vi "Vision_Init.vi"(10 "Front Panel.WinBounds":T1, 11 "Refnum in":T2="cam1") -> (0 "error out":errorcluster, 1 "Image (duplicate)":T4, 2 "Object Tracking Session Out":T5, 3 "Refnum out":T2, 4 "Center Point":T3)   [LabVIEW 2017]
doc: "This VI configures a USB camera for frame grabbing, and sets up the first image with the Traditional MeanShift tracking algorithm. Select the center point of the image, and place a rectangle around the region of interest to set up tracking."
uses:
  <vilib>/userdefined/High Color/IMAQdx.ctl
  <vilib>/vision/Tracking.llb/IMAQ Object Tracking Session.ctl
  <vilib>/vision/Image Controls.llb/IMAQ Image.ctl
  <vilib>/Utility/miscctls.llb/LVRectTypeDef.ctl
  <vilib>/vision/driver/NI_Vision_Acquisition_Software.lvlib
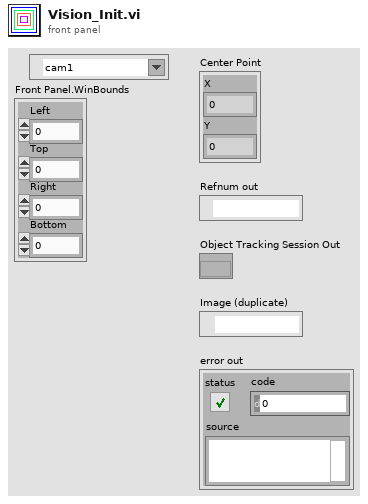
[diagram p1: front panel]
types:
  T1 = typedef "LVRectTypeDef.ctl" = cluster{"Left":i16, "Top":i16, "Right":i16, "Bottom":i16}
  T2 = typedef "IMAQdx.ctl" = refnum<k21>
  T3 = typedef "IMAQ Point" = cluster{"X":sgl, "Y":sgl}
  T4 = typedef "IMAQ Image.ctl" = refnum<image>
  T5 = typedef "IMAQ Object Tracking Session.ctl" = refnum<k20>
  T6 = typedef "Image Type" = u32
  T7 = cluster{"Number of Histogram Bins":i32, "Blending Parameter (%)":dbl, "Maximum Iterations":i32}
  T8 = typedef "ROI Descriptor" = cluster{"Global Rectangle":i32[], "Contours":cluster{"ID":enum32{"External", "Internal"}, "Type":u32, "Coordinates":i32[]}[]}
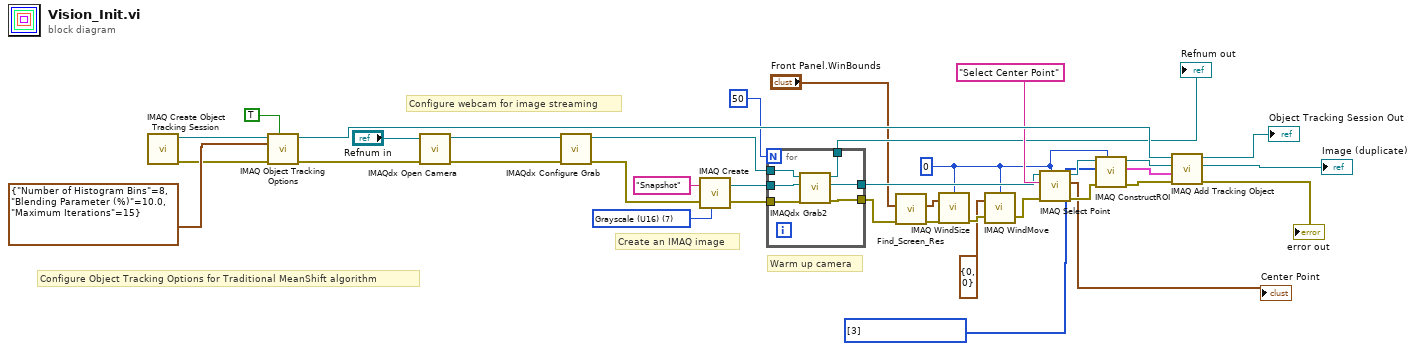
[diagram p0: block diagram]
diagram:
  w2 = 0 ("Window Number")
  w32 = u32[] [3] items=["No Selection", "Point", "Line", "Rectangle", "Oval", "Polygon", "Freehand Region", "Annulus", "Zoom", "Pan", "Broken Line", "Freehand Line", "Rotated Rectangle"] ("Tools")
  w15 = T6 7 items=["Grayscale (U8)", "Grayscale (I16)", "Grayscale (SGL)", "Complex (CSG)", "RGB (U32)", "HSL (U32)", "RGB (U64)", "Grayscale (U16)"] ("Image Type")
  # "Warm up camera"
  # "Create an IMAQ image"
  # "Configure webcam for image streaming"
  # "Configure Object Tracking Options for Traditional MeanShift algorithm"
  n1 = call "IMAQ Create Object Tracking Session"() -> ("error out"=w12:errorcluster, "Object Tracking Session"=w10:T5)  [unwired: 1 in, 9 out]
  n2 = call-poly "IMAQ Object Tracking Options"("Get/Set (Get)"=TRUE, "error in (no error)"=w12, "Mean Shift Options in"=T7 {"Number of Histogram Bins"=8, "Blending Parameter (%)"=10.0, "Maximum Iterations"=15}, "Object Tracking Session In"=w10) -> ("error out"=w16:errorcluster, "Object Tracking Session Out"=w37:T5)  [unwired: 5 in, 1 out]
  n3 = call <vilib>:"IMAQdx Open Camera.vi"("error in"=w16, "Session In"="Refnum in") -> ("error out"=w18:errorcluster, "Session Out"=w17:T2)  [unwired: 8 in]
  n4 = call <vilib>:"IMAQdx Configure Grab.vi"("error in"=w18, "Session In"=w17) -> ("error out"=w19:errorcluster, "Session Out"=w21:T2)  [unwired: 8 in]
  n5 = call "IMAQ Create"("Image Name"="Snapshot", "Image Type"=w15, "error in (no error)"=w19) -> ("New Image"=w22:T4, "error out"=w23:errorcluster)  [unwired: 2 in]
  n6 = for {
    N: 50 -> [_]
    tunnel: w21 -> [w43]
    tunnel: w22 -> [w42]
    tunnel: w23 -> [w41]
    tunnel: [w40] -> w8
    tunnel: [w39] -> w25
    tunnel: [w38] -> w24
    n7 = call <vilib>:"IMAQdx Grab2.vi"("error in"=w41, "Image In"=w42, "Session In"=w43) -> ("error out"=w40:errorcluster, "Image Out"=w39:T4, "Session Out"=w38:T2)  [unwired: 5 in, 1 out]
  }
  "Refnum out" <- w24
  n8 = call "Find_Screen_Res.vi"("error in (no error)"=w8, "Front Panel.WinBounds"="Front Panel.WinBounds") -> ("error out"=w7:errorcluster, "Width & Height"=w6:cluster{"Width":i32, "Height":i32})  [unwired: 8 in]
  n9 = call "IMAQ WindSize"("error in (no error)"=w7, "Width & Height"=w6, "Window Number"=w2) -> ("error out"=w5:errorcluster)  [unwired: 3 in, 2 out]
  n10 = call "IMAQ WindMove"("Window Number (0...15)"=w2, "Coordinates (screen)"=cluster{"X Position":i32, "Y Position":i32} {"X Position"=0, "Y Position"=0}, "error in (no error)"=w5) -> ("error out"=w4:errorcluster)  [unwired: 2 in, 1 out]
  n11 = call "IMAQ Select Point"("Window Number (0...15)"=w2, "error in (no error)"=w4, "Prompt"="Select Center Point", "Image In"=w25) -> ("error out"=w33:errorcluster, "Point"=→"Center Point":T3, "Image Out (duplicate)"=w34:T4)  [unwired: 4 in, 1 out]
  n12 = call "IMAQ ConstructROI"("Window Number (-1...15)"=w2, "error in (no error)"=w33, "Tools"=w32, "Image"=w34) -> ("error out"=w31:errorcluster, "ROI Descriptor Out"=w30:T8, "Image Out (duplicate)"=w29:T4)  [unwired: 4 in, 1 out]
  n13 = call "IMAQ Add Tracking Object"("error in (no error)"=w31, "ROI Descriptor"=w30, "Image"=w29, "Object Tracking Session In"=w37) -> ("error out"=→"error out":errorcluster, "Image (duplicate)"=→"Image (duplicate)":T4, "Object Tracking Session Out"=→"Object Tracking Session Out":T5)  [unwired: 1 in, 4 out]
